vi "zmq timers cancel.vi"(8 "error in (no error)":errorcluster, 10 "timer_id":i32, 11 "timers":u32) -> (0 "error out":errorcluster, 2 "function return":i32, 3 "timers out":u32)   [LabVIEW 2025, in "LibZMQ.lvlib"]
doc: "ZMQ_EXPORT int zmq_timers_cancel (void *timers, int timer_id);"
uses:
  LibZMQ.lvlib
  LV/LibZMQ/libzmq/lv_x86/bin/Release/libzmq-v143-mt-4_3_6.dll
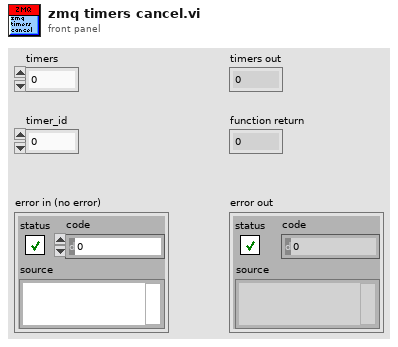
[diagram p1: front panel]
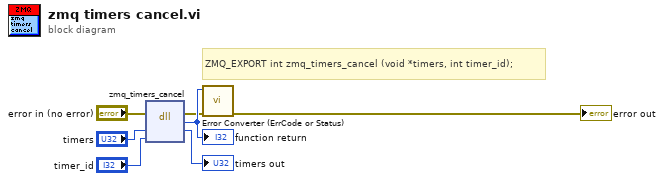
[diagram p0: block diagram]
diagram:
  # "ZMQ_EXPORT int zmq_timers_cancel (void *timers, int timer_id);"
  n1 = dll-call lib="C:/LV/LibZMQ/libzmq/lv_x86/bin/Release/libzmq-v143-mt-4_3_6.*" fn="zmq_timers_cancel"(error in="error in (no error)", "timers"="timers", "timer_id"="timer_id") -> (error out=w2:errorcluster, w7:i32, "timers"=→"timers out":u32)  [unwired: 3 in, 1 out]
  "function return" <- w7
  n2 = call "Error Converter (ErrCode or Status).vi"("error in (no error)"=w2, "error code"=w7) -> ("error out"=→"error out":errorcluster)  [unwired: 9 in]
